vi "ASK.vi"() -> ()   [LabVIEW 2009]
doc: "For a square root raised cosine pulse shape, you end up with a raised cosine pulse shape here. Raised cosine pulse shape,\nyou end up with a square of a raised cosine pulse shape (which isn't a Nyquist pulse). Triangle waves for no pulse shaping\n(rectangular pulses). Sample at integer multiples of the symbol period and see if that sample is closer to zero or closer to\nsqrt(0.002) to determine if it is a zero or one (maximum likelihood detection)."
uses:
  <vilib>/addons/Modulation/Analog/MT Downconvert Passband (Real).vi
  <vilib>/addons/Modulation/Analog/MT Upconvert Baseband (Real).vi
  <vilib>/addons/Modulation/Digital/General/MT Generate Bits (Galois, PN Order).vi
  <vilib>/addons/Spectral Measurements Toolset/LVSupport/SMT Basic Zoom Power Spectrum (WDT).vi
  <vilib>/measure/macond.llb/FIR Filter for 1 Chan.vi
  Instance          14 16Saved   ASK-rev2 .vi
  <vilib>/measure/NI_MAPro.lvlib
panel:
  in  "Tab Control":T1(tab)
  out "Passband time domain signal (delayed due to group delay of passband filter)":waveform(dbl)(graph)={"t0"=timestamp(0 s since 1904-01-01), "dt"=5e-10, "Y"=[]}
  out "Pulse Shaped Baseband Signal":waveform(dbl)(graph)={"t0"=timestamp(0 s since 1904-01-01), "dt"=5e-10, "Y"=[]}
  out "Normalized (Peak Signal Power = 0 dBm) Power Spectrum (Average over one block of bits)":cluster{"f0":dbl, "df":dbl, "spectrum":dbl[]}(graph)={"f0"=2499999.9999999995, "df"=2499999.9999999995, "spectrum"=[]}
  out "Recovered Baseband Signal (After matched filtering and downsampling)":waveform(dbl)(graph)={"t0"=timestamp(0 s since 1904-01-01), "dt"=5e-10, "Y"=[]}
  in  "Random Pattern / 101010 Pattern":bool
  in  "modulation type 2":enum16{"FSK", "PSK", "QAM", "MSK", "PAM", "ASK"}(ring)=enum."PAM"
  in  "Delay per cycle (Seconds)":dbl=1.0 caption="Delay Time (s)"
  in  "optional FIR filter specifications":T2={"PB Gain"=0.0, "SB Gain"=-60.0, "Scale"=TRUE, "Window"=enum."Flat Top"} {"SB Gain" format="%.2p"; "PB Gain" format="%.2p"}
  out "Symbol Period":dbl=2.5e-08
  out "Number of Bit Errors":i8
  in  "Eb/N0 (dB)":dbl=9000.0 format="%.2f"
  out "Decoded Bits (16 shown at a time, scroll to view remainder)":i8[](array[numeric])=[1, 0, 1, 1, 0, 1, 1, 1, 1, 1, 1, 0, 0, 0, 0, 1, 1, 0, 1, 1, 0, 0, 0, 0, 0, 1, 0, 0, 0, 1, 0, 1, 1, 0, 1, 0, 0, 0, 0, 1, 1, 0, 0, 1, 1, 1, 0, 1, 1, 1, 0, 0, 0, 1, 0, 1, 0, 1, 0, 0, 1, 1, 0, 0, 1, 0, 0, 1, 1, 1, 1, 1, 1, 0, 1, 0, 1, 0, 1, 1, 0, 1, 0, 0, 0, 0, 0, 1, 1, 1, 1, 1, 1, 0, 1, 1, 1, 0, 0, 0, 0, 1, 0, 0, 0, 0, 0, 1, 1, 0, 0, 1, 0, 0, 0, 1, 1, 0, 0, 0, 0, 1, 0, 1]
  in  "unit conversion settings":T3={"units"=enum."dBm", "peak scaling"=enum."rms", "psd?"=FALSE, "impedance(ohm)"=1.0} {"impedance(ohm)" format="%.2f"}
  out "Signal Bandwidth":dbl=20000000.0 format="%#.6p"
  in  "Filter parameter (Rolloff Factor)":dbl=1.0 format="%.2f"
  in  "Carrier Frequency (Hz)":dbl=1000000000.0 min=-0.5 max=0.5 format="%#.6p"
  in  "modulation type":enum16{"FSK", "PSK", "QAM", "MSK", "PAM", "ASK"}(ring)=enum."ASK"
  in  "pulse shaping filter (none)":T4(ring)=enum."Root Raised Cos"
  in  "filter length (symbols)":i32=8
  in  "Symbol Rate (Hz)":dbl=30000000.0 format="%#.6p"
  in  "Terminate Simulation":bool
  out "Bits (16 shown at a time, scroll to view remainder of stream)":i8[](array[numeric])=[1, 0, 1, 1, 0, 1, 1, 1, 1, 1, 1, 0, 0, 0, 0, 1, 1, 0, 1, 1, 0, 0, 0, 0, 0, 1, 0, 0, 0, 1, 0, 1, 1, 0, 1, 0, 0, 0, 0, 1, 1, 0, 0, 1, 1, 1, 0, 1, 1, 1, 0, 0, 0, 1, 0, 1, 0, 1, 0, 0, 1, 1, 0, 0, 1, 0, 0, 1, 1, 1, 1, 1, 1, 0, 1, 0, 1, 0, 1, 1, 0, 1, 0, 0, 0, 0, 0, 1, 1, 1, 1, 1, 1, 0, 1, 1, 1, 0, 0, 0, 0, 1, 0, 0, 0, 0, 0, 1, 1, 0, 0, 1, 0, 0, 0, 1, 1, 0, 0, 0, 0, 1, 0, 1, 0, 1, 1, 0]
  in  "PN sequence order (Valid range 6-15)":i32=6 min=5 max=31
  in  "Number of Bits to Generate":i32=128
  in  "Bit Sequence Generation Type  (Galois PN, Uniform Random)":bool
  # "Configuration"
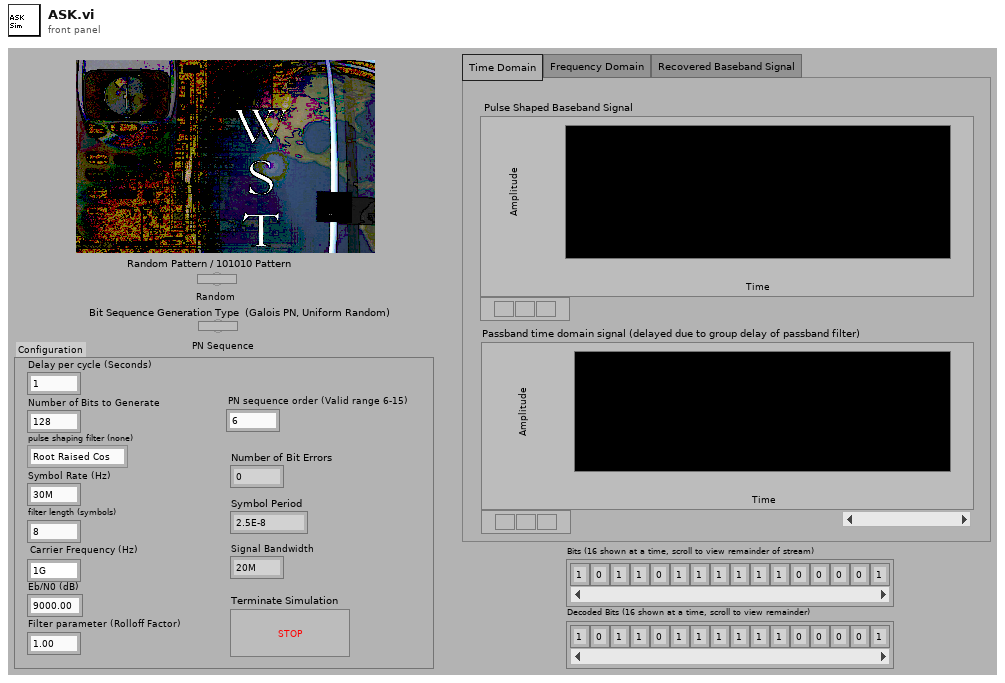
[diagram p1: front panel]
types:
  T1 = enum32{"Time Domain", "Frequency Domain", "Recovered Baseband Signal"}
  T2 = cluster{"PB Gain":dbl, "SB Gain":dbl, "Scale":bool, "Window":enum16{"None", "Hanning", "Hamming", "Triangular", "Blackman", "Exact Blackman", "Blackman-Harris", "Kaiser-Bessel", "Flat Top"}}
  T3 = cluster{"units":enum16{"V", "V^2", "W", "dBm", "dBW", "dBV", "dBmV", "dBuV"}, "peak scaling":enum16{"rms", "pk"}, "psd?":bool, "impedance(ohm)":dbl}
  T4 = enum16{"none", "Raised Cosine", "Root Raised Cos"}
  T5 = cluster{"Topology":enum16{"Off", "FIR by Specification", "Equi-ripple FIR", "Windowed FIR"}, "Type":enum16{"Lowpass", "Highpass", "Bandpass", "Bandstop"}, "#Taps":i32, "Lower PB":dbl, "Upper PB":dbl, "Lower SB":dbl, "Upper SB":dbl}
  T6 = enum16{"Lowpass", "Highpass", "Bandpass", "Bandstop"}
  T7 = enum16{"Off", "FIR by Specification", "Equi-ripple FIR", "Windowed FIR"}
  T8 = enum16{"none", "Raised Cosine", "Root Raised Cos", "Gaussian"}
  T9 = typedef "Complex Data Waveform.ctl" = cluster{"t0":dbl, "dt":dbl, "Y":cdb[]}
  T10 = cluster{"spectrum type":enum16{"FFT Spectrum [complex]", "Amplitude [Magnitude]", "Power [Magnitude^2]", "Cross Spectrum [complex]", "Frequency Response [Complex]"}, "linear/dB":enum16{"linear", "dB"}, "window":enum16{"None ", "Hanning", "Hamming", "Blackman-Harris", "Exact Blackman", "Blackman", "Flat Top", "4 Term B-Harris ", "7 Term B-Harris", "Low Sidelobe"}, "window size":i32, "FFT size":i32}
  T11 = typedef "NI_MAPro.lvlib/ma_sml_Spectrum Cluster (real).ctl" = cluster{"f0":dbl, "df":dbl, "spectrum":dbl[]}
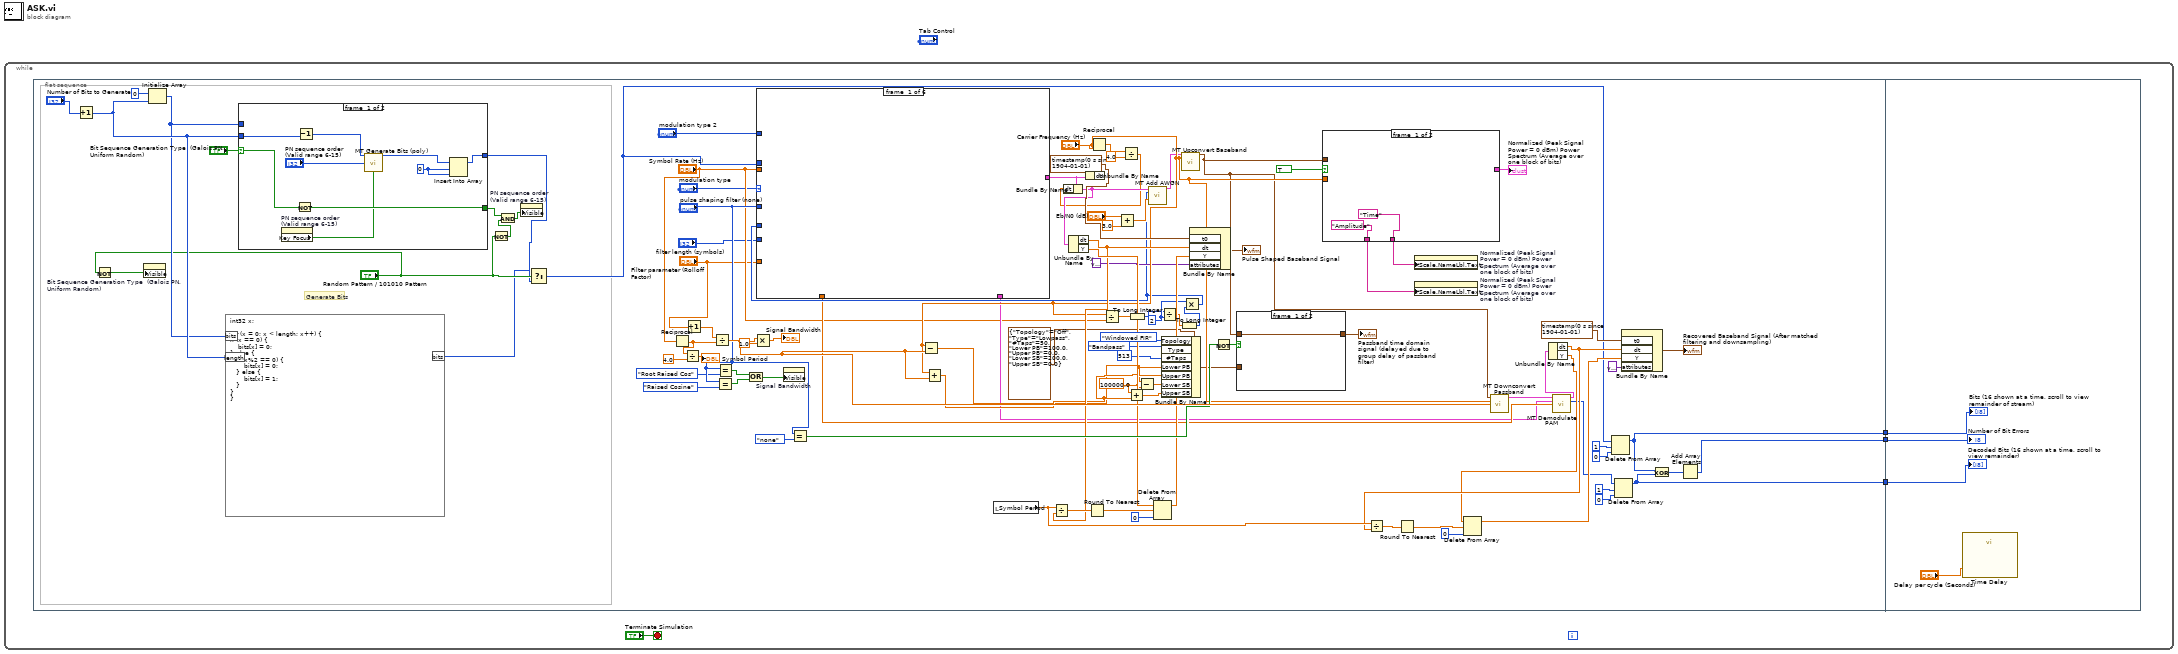
[diagram p0: block diagram]
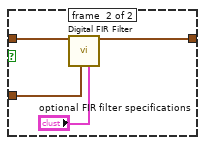
[diagram p2: hidden frame]
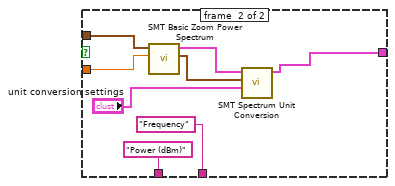
[diagram p3: hidden frame]
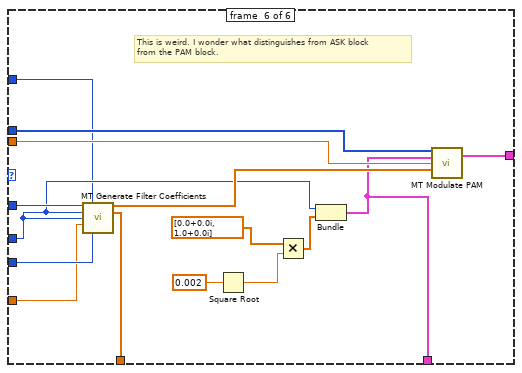
[diagram p8: hidden frame]
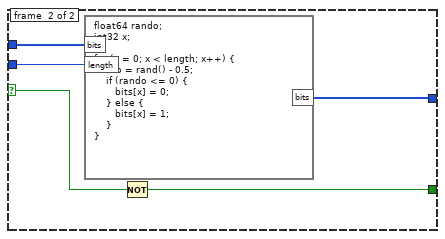
[diagram p9: hidden frame]
diagram:
  n1 = while {
    stop <- "Terminate Simulation" stop-if-true
    n2 = flat-sequence {
      tunnel: [w15] -> w3
      tunnel: [w14] -> w2
      tunnel: [w13] -> w1
      tunnel: w3 -> [w149]
      tunnel: w2 -> [w148]
      tunnel: w1 -> [w147]
      frame #0 {
        w63 = 100000.0 ("Lower SB")
        w36 = 2 ("y")
        # "Generate Bits"
        n3 = Increment(x="Number of Bits to Generate") -> (x+1=w101:i32)
        n4 = Not(x="Random Pattern / 101010 Pattern") -> (.not. x?=w12:bool)
        n5 = property on="Bit Sequence Generation Type  (Galois PN, Uniform Random)" class="Bool (strict)"("Visible"=w12) -> ()  [unwired: 2 in, 2 out]
        n6 = Initialize Array(i8 0, w101) -> (w100:i8[])
        n7 = formula code="int32 x;\n\nfor (x = 0; x < length; x++) {\nif (x == 0) {\n    bits[x] = 0;\n} else {\n   if (x%2 == 0) {\n       bits[x] = 0;\n   } else {\n       bits[x] = 1;\n   }\n}\n}"("bits"=w100, "length"=w101) -> ("bits"=w5:i8[])
        n8 = case shown="True" "Bit Sequence Generation Type  (Galois PN, Uniform Random)" {
          selector: "Bit Sequence Generation Type  (Galois PN, Uniform Random)" -> [w140 w143]
          tunnel: w101 -> [w137 w145]
          tunnel: [w133 w144] -> w6
          tunnel: w100 -> [_ w146]
          tunnel: [w139 w142] -> w9
          frame #0 {
            w135 = 0 ("index")
            n9 = property on="PN sequence order (Valid range 6-15)" class="DigNum (strict)"() -> ("Key Focus"=w138:bool)  [unwired: 2 in, 2 out]
            n10 = Not(x=w140) -> (.not. x?=w139:bool)
            n11 = Decrement(x=w137) -> (x-1=w136:i32)
            n12 = call-poly <vilib>:"MT Generate Bits (poly).vi"("total bits (128)"=w136, "PN sequence order (9)"="PN sequence order (Valid range 6-15)", "reset? (T)"=w138) -> ("output bit stream"=w134:i8[])  [unwired: 10 in, 2 out]
            n13 = Insert Into Array(array=w134, index=w135, new element=w135) -> (w133:i8[])
          }
          frame #1 {
            n14 = formula code="float64 rando;\nint32 x;\n\nfor (x = 0; x < length; x++) {\nrando = rand() - 0.5;\n    if (rando <= 0) {\n       bits[x] = 0;\n    } else {\n       bits[x] = 1;\n    }\n}"("bits"=w146, "length"=w145) -> ("bits"=w144:i8[])
            n15 = Not(x=w143) -> (.not. x?=w142:bool)
          }
        }
        n16 = Not(x="Random Pattern / 101010 Pattern") -> (.not. x?=w10:bool)
        n17 = And(x=w9, y=w10) -> (x .and. y?=w8:bool)
        n18 = property on="PN sequence order (Valid range 6-15)" class="DigNum (strict)"("Visible"=w8) -> ()  [unwired: 2 in, 2 out]
        n19 = Select(t=w5, s="Random Pattern / 101010 Pattern", f=w6) -> (s? t:f=w7:i8[])
        n20 = Reciprocal(x="Symbol Rate (Hz)") -> (1/x=w66:dbl)
        n21 = Divide(x=w66, y=4.0) -> (x/y=→"Symbol Period":dbl)
        n22 = Increment(x="Filter parameter (Rolloff Factor)") -> (x+1=w21:dbl)
        n23 = Divide(x=w21, y=w66) -> (x/y=w95:dbl)
        n24 = Equal?(x="pulse shaping filter (none)", y=T8."Raised Cosine") -> (x = y?=w23:bool)
        n25 = Equal?(x="pulse shaping filter (none)", y=T8."Root Raised Cos") -> (x = y?=w22:bool)
        n26 = Or(x=w22, y=w23) -> (x .or. y?=w90:bool)
        n27 = Multiply(x=w95, y=1.0) -> (x*y=→"Signal Bandwidth":dbl)
        n28 = property on="Signal Bandwidth" class="DigNum (strict)"("Visible"=w90) -> ()  [unwired: 2 in, 2 out]
        n29 = Equal?(x="pulse shaping filter (none)", y=T4."none") -> (x = y?=w93:bool)
        n30 = Subtract(x="Carrier Frequency (Hz)", y=w95) -> (x-y=w61:dbl)
        n31 = Add(x="Carrier Frequency (Hz)", y=w95) -> (x+y=w64:dbl)
        n32 = local read "Symbol Period"() -> (w87:dbl)
        n33 = Reciprocal(x="Carrier Frequency (Hz)") -> (1/x=w26:dbl)
        n34 = Divide(x="Carrier Frequency (Hz)", y="Symbol Rate (Hz)") -> (x/y=w34:dbl)
        n35 = Add(x="Eb/N0 (dB)", y=3.0) -> (x+y=w99:dbl)
        n36 = Divide(x=w26, y=4.0) -> (x/y=w32:dbl)
        n37 = Add(x=w63, y=w64) -> (x+y=w62:dbl)
        n38 = To Long Integer(number=w34) -> (32bit integer=w35:i32)
        n39 = Subtract(x=w61, y=w63) -> (x-y=w60:dbl)
        n40 = Divide(x=w35, y=w36) -> (x/y=w37:dbl)
        n41 = Bundle By Name(cluster=T5 {"Topology"=enum."Off", "Type"=enum."Lowpass", "#Taps"=50, "Lower PB"=100.0, "Upper PB"=0.0, "Lower SB"=200.0, "Upper SB"=0.0} ("FIR filter specifications"), "Topology"=T7."Windowed FIR", "Type"=T6."Bandpass", "#Taps"=513, "Lower PB"=w61, "Upper PB"=w64, "Lower SB"=w60, "Upper SB"=w62) -> (w58:T5)
        n42 = To Long Integer(number=w37) -> (32bit integer=w38:i32)
        n43 = Multiply(x=w36, y=w38) -> (x*y=w43:i32)
        n44 = case shown="\"ASK\"" "modulation type" {
          tunnel: "Symbol Rate (Hz)" -> [_ _ _ _ _ w131]
          tunnel: "filter length (symbols)" -> [_ _ _ _ _ w130]
          tunnel: "pulse shaping filter (none)" -> [_ _ _ _ _ w129]
          tunnel: w7 -> [_ _ _ _ _ w128]
          tunnel: [_ _ _ _ _ w127] -> w45
          tunnel: "Filter parameter (Rolloff Factor)" -> [_ _ _ _ _ w126]
          tunnel: w43 -> [_ _ _ _ _ w125]
          tunnel: [_ _ _ _ _ w124] -> w40
          tunnel: [_ _ _ _ _ w123] -> w41
          tunnel: "modulation type 2" -> [_ _ _ _ _ w118]
          frame #0 {
          }
          frame #1 {
          }
          frame #2 {
          }
          frame #3 {
          }
          frame #4 {
          }
          frame #5 {
            # "This is weird. I wonder what distinguishes from ASK block\nfrom the PAM block."
            n45 = call <vilib>:"MT Generate Filter Coefficients.vi"("pulse shaping filter (none)"=w129, "modulation type"=w118, "pulse shaping samples per symbol (16)"=w125, "matched samples per symbol (16)"=w125, "filter parameter"=w126, "filter length (symbols)"=w130) -> ("pulse shaping filter coefficients"=w132:dbl[], "matched filter coefficients"=w123:dbl[])  [unwired: 7 in, 1 out]
            n46 = Square Root(x=0.002) -> (sqrt(x)=w120:dbl)
            n47 = Multiply(x=cdb[] [0.0+0.0i, 1.0+0.0i] ("symbol map"), y=w120) -> (x*y=w119:cdb[])
            n48 = Bundle(w125, w119) -> (w124:cluster{i32, cdb[]})  [unwired: 1 in]
            n49 = call <vilib>:"MT Modulate PAM.vi"("input bit stream"=w128, "PAM system parameters"=w124, "symbol rate (Hz)"=w131, "pulse shaping filter coefficients"=w132) -> ("output complex waveform"=w127:T9)  [unwired: 9 in, 2 out]
          }
        }
        n50 = Bundle By Name(cluster=w45, "dt"=w32) -> (w46:T9)
        n51 = Unbundle By Name(w46) -> ("dt"=w76:dbl, "Y"=w80:cdb[])
        n52 = Divide(x=w87, y=w76) -> (x/y=w77:dbl)
        n53 = Unbundle By Name(w45) -> ()  [unwired: 1 out]
        n54 = Round To Nearest(number=w77) -> (nearest integer value=w79:dbl)
        n55 = call <vilib>:"MT Add AWGN.vi"("input complex waveform"=w46, "samples per symbol (16)"=w43, "Eb/N0 (10 dB)"=w99) -> ("output complex waveform"=w42:T9)  [unwired: 10 in, 2 out]
        n56 = Delete From Array(array=w80, length=w79, index=0) -> (array with subset deleted=w81:cdb[])  [unwired: 1 out]
        n57 = call-poly <vilib>:"MT Upconvert Baseband.vi"("baseband waveform (complex)"=w42, "carrier frequency (Hz)"="Carrier Frequency (Hz)") -> ("passband waveform"=w52:waveform(dbl))  [unwired: 12 in, 1 out]
        n58 = Bundle By Name("t0"=timestamp(0 s since 1904-01-01), "dt"=w76, "Y"=w81, "attributes"=variant) -> (→"Pulse Shaped Baseband Signal":waveform(cdb))  [unwired: 1 in]
        n59 = Not(x=w93) -> (.not. x?=w89:bool)
        n60 = case shown="True" w89 {
          tunnel: w52 -> [w103 w107]
          tunnel: [w103 w106] -> w53
          tunnel: w58 -> [_ w104]
          frame #0 {
          }
          frame #1 {
            n61 = call-poly <vilib>:"Digital FIR Filter.vi"("optional FIR filter specifications"="optional FIR filter specifications", "FIR filter specifications"=w104, "signal in"=w107) -> ("signal out"=w106:waveform(dbl))  [unwired: 6 in, 2 out]
          }
        }
        "Passband time domain signal (delayed due to group delay of passband filter)" <- w53
        n62 = case shown="True" TRUE {
          tunnel: w52 -> [_ w114]
          tunnel: "Carrier Frequency (Hz)" -> [_ w117]
          tunnel: ["Time" ("X Scale.Name Label.Text") "Frequency" ("X Scale.Name Label.Text")] -> w28
          tunnel: ["Amplitude" ("X Scale.Name Label.Text") "Power (dBm)" ("X Scale.Name Label.Text")] -> w29
          tunnel: [_ w110] -> w30
          frame #0 {
          }
          frame #1 {
            n63 = call-poly <vilib>:"SMT Basic Zoom Power Spectrum.vi"("center frequency"=w117, "signal in"=w114) -> ("spectral info"=w112:T10, "power spectrum"=w113:T11)  [unwired: 6 in, 2 out]
            n64 = call <vilib>:"SMT Spectrum Unit Conversion.vi"("unit conversion settings"="unit conversion settings", "spectral info in"=w112, "power spectrum"=w113) -> ("unit converted spectrum"=w110:cluster{"f0":dbl, "df":dbl, "spectrum":dbl[]})  [unwired: 5 in, 3 out]
          }
        }
        "Normalized (Peak Signal Power = 0 dBm) Power Spectrum (Average over one block of bits)" <- w30
        n65 = property on="Normalized (Peak Signal Power = 0 dBm) Power Spectrum (Average over one block of bits)" class="WFGraph (strict)"("XScale.NameLbl.Text"=w28) -> ()  [unwired: 2 in, 2 out]
        n66 = property on="Normalized (Peak Signal Power = 0 dBm) Power Spectrum (Average over one block of bits)" class="WFGraph (strict)"("YScale.NameLbl.Text"=w29) -> ()  [unwired: 2 in, 2 out]
        n67 = call-poly <vilib>:"MT Downconvert Passband.vi"("Waveform"=w52, "carrier frequency (Hz)"="Carrier Frequency (Hz)", "passband bandwidth (Hz)"=w95) -> ("downconverted waveform (complex baseband)"=w39:T9)  [unwired: 9 in, 3 out]
        n68 = call <vilib>:"MT Demodulate PAM.vi"("input complex waveform"=w39, "PAM system parameters"=w40, "matched filter coefficients"=w41) -> ("recovered complex waveform"=w49:T9, "output bit stream"=w73:i8[])  [unwired: 8 in, 3 out]
        n69 = Unbundle By Name(w49) -> ("dt"=w86:dbl, "Y"=w85:cdb[])
        n70 = Divide(x=w87, y=w86) -> (x/y=w82:dbl)
        n71 = Round To Nearest(number=w82) -> (nearest integer value=w83:dbl)
        n72 = Delete From Array(array=w85, length=w83, index=0) -> (array with subset deleted=w88:cdb[])  [unwired: 1 out]
        n73 = Delete From Array(array=w7, length=1, index=0) -> (array with subset deleted=w15:i8[])  [unwired: 1 out]
        n74 = Delete From Array(array=w73, length=1, index=0) -> (array with subset deleted=w14:i8[])  [unwired: 1 out]
        n75 = Bundle By Name("t0"=timestamp(0 s since 1904-01-01), "dt"=w86, "Y"=w88, "attributes"=variant) -> (→"Recovered Baseband Signal (After matched filtering and downsampling)":waveform(cdb))  [unwired: 1 in]
        n76 = Exclusive Or(1:w14, 2:w15) -> (0:w44:i8[])
        n77 = Add Array Elements(numeric array=w44) -> (sum=w13:i8)
      }
      frame #1 {
        n78 = call "Time Delay"("Delay Time (s)"="Delay per cycle (Seconds)") -> ()  [unwired: 10 in, 1 out]
        "Bits (16 shown at a time, scroll to view remainder of stream)" <- w149
        "Decoded Bits (16 shown at a time, scroll to view remainder)" <- w148
        "Number of Bit Errors" <- w147
      }
    }
  }
